vi "Get Discovery Service Address.vi"(8 "error in":errorcluster, 11 "cluster id (\"\")":string) -> (0 "error out":errorcluster, 3 "address":string)   [LabVIEW 2020, in "NI Discovery V1 Client.lvlib"]
uses:
  NI Discovery V1 Client.lvlib
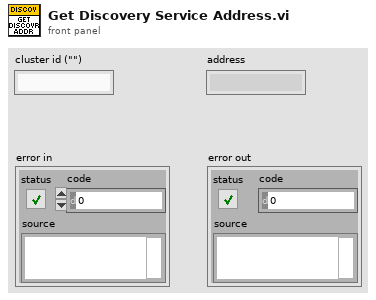
[diagram p1: front panel]
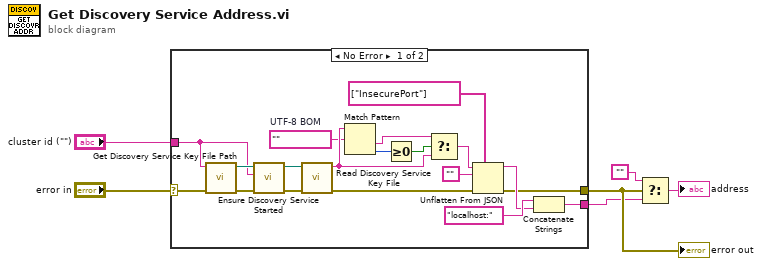
[diagram p0: block diagram]
diagram:
  n1 = case shown="No Error" "error in" {
    selector: "error in" -> [w8 w26]
    tunnel: "cluster id (\"\")" -> [w7 _]
    tunnel: [w14 w26] -> w5
    tunnel: [w13 _] -> w3
    frame No Error {
      w19 = "﻿"  # UTF-8 BOM
      n2 = call "Get Discovery Service Key File Path.vi"("error in"=w8, "cluster id (\"\")"=w7) -> ("error out"=w12:errorcluster, "key file path"=w10:path)  [unwired: 8 in]
      n3 = call "Ensure Discovery Service Started.vi"("error in"=w12, "cluster id"=w7, "path"=w10) -> ("error out"=w11:errorcluster, "key file path"=w9:path)  [unwired: 7 in]
      n4 = call "Read Discovery Service Key File.vi"("error in"=w11, "key file path"=w9) -> ("error out"=w17:errorcluster, "key json"=w20:string)  [unwired: 8 in]
      n5 = Match Pattern(string=w20, regular expression=w19) -> (after substring=w23:string, offset past match=w22:i32)  [unwired: 1 in, 2 out]
      n6 = Greater Or Equal To 0?(x=w22) -> (x >= 0?=w24:bool)
      n7 = Select(t=w23, s=w24, f=w20) -> (s? t:f=w25:string)
      n8 = Unflatten From JSON(path=string[] ["InsecurePort"], JSON string=w25, type and defaults="", error in (no error)=w17) -> (value=w15:string, error out=w14:errorcluster)  [unwired: 3 in]
      n9 = Concatenate Strings("localhost:", w15) -> (w13:string)
    }
    frame Error {
    }
  }
  "error out" <- w5
  n10 = Select(t="", s=w5, f=w3) -> (s? t:f=→"address":string)
